vi "Set Conditional Symbols.vi"(0 "Project Path":path, 2 "w_visa":bool, 3 "w_daqmx":bool, 11 "error in (no error)":errorcluster) -> (15 "error out":errorcluster)   [LabVIEW 2013]
doc: "VI sets conditional symbols in the project."
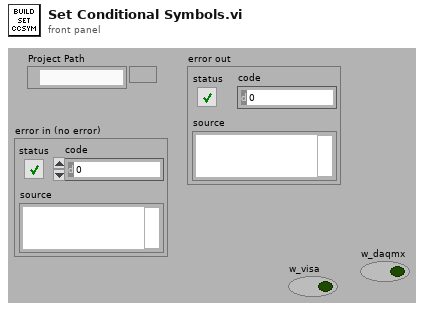
[diagram p1: front panel]
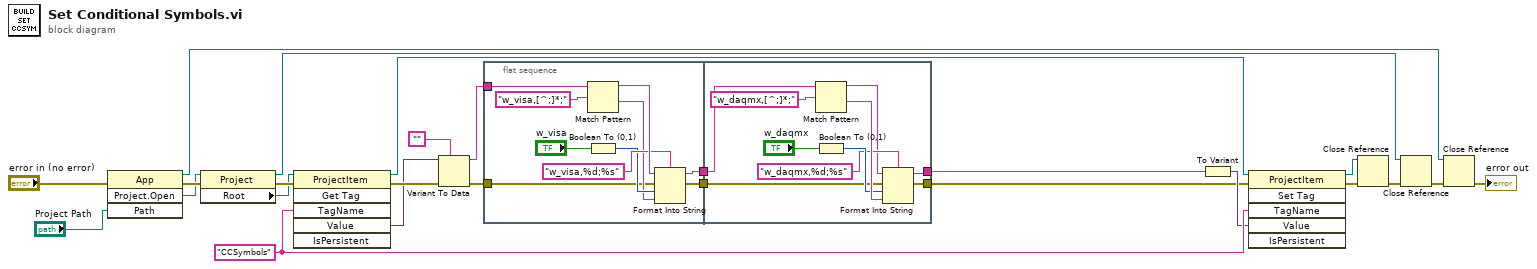
[diagram p0: block diagram]
diagram:
  w22 = "CCSymbols" ("Tag Name")
  n1 = invoke class="App" method="Project.Open"(error in="error in (no error)", "Path"="Project Path") -> (reference out=w13:refnum<vi>, error out=w14:errorcluster, "Project:Open"=w11:refnum<vi>)  [unwired: 2 in, 1 out]
  n2 = property class="Project"(reference=w11, error in=w14) -> (reference out=w12:refnum<vi>, error out=w21:errorcluster, "Root"=w6:refnum<vi>)
  n3 = invoke class="ProjectItem" method="Get Tag"(reference=w6, error in=w21, "TagName"=w22) -> (reference out=w5:refnum<vi>, error out=w24:errorcluster, "Value"=w23:variant)  [unwired: 3 in, 3 out]
  n4 = Variant To Data(error in=w24, type="", Variant=w23) -> (data=w1:string, error out=w2:errorcluster)
  n5 = flat-sequence {
    tunnel: [w29] -> w4
    tunnel: [w28] -> w3
    tunnel: w2 -> [w27]
    tunnel: w1 -> [w26]
    tunnel: [w38] -> w8
    tunnel: [w37] -> w10
    tunnel: w4 -> [w36]
    tunnel: w3 -> [w39]
    frame #0 {
      n6 = Match Pattern(string=w26, regular expression="w_visa,[^;]*;") -> (before substring=w34:string, after substring=w30:string)  [unwired: 1 in, 2 out]
      n7 = Boolean To (0,1)(Boolean="w_visa") -> (0, 1=w31:i16)
      n8 = Format Into String(format string="w_visa,%d;%s", initial string=w34, error in=w27, w31, w30) -> (resulting string=w29:string, error out=w28:errorcluster)
    }
    frame #1 {
      n9 = Match Pattern(string=w36, regular expression="w_daqmx,[^;]*;") -> (before substring=w41:string, after substring=w45:string)  [unwired: 1 in, 2 out]
      n10 = Boolean To (0,1)(Boolean="w_daqmx") -> (0, 1=w44:i16)
      n11 = Format Into String(format string="w_daqmx,%d;%s", initial string=w41, error in=w39, w44, w45) -> (resulting string=w37:string, error out=w38:errorcluster)
    }
  }
  n12 = To Variant(anything=w10) -> (Variant=w9:variant)
  n13 = invoke class="ProjectItem" method="Set Tag"(reference=w5, error in=w8, "TagName"=w22, "Value"=w9) -> (reference out=w18:refnum<vi>, error out=w17:errorcluster)  [unwired: 2 in, 4 out]
  n14 = Close Reference(reference=w18, error in (no error)=w17) -> (error out=w15:errorcluster)
  n15 = Close Reference(reference=w12, error in (no error)=w15) -> (error out=w16:errorcluster)
  n16 = Close Reference(reference=w13, error in (no error)=w16) -> (error out=→"error out":errorcluster)
